vi "Latch.vi"(1 "Reset":bool, 2 "In":bool) -> (0 "Out":bool)   [LabVIEW 2013]
panel:
  in  "var":bool
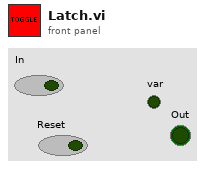
[diagram p1: front panel]
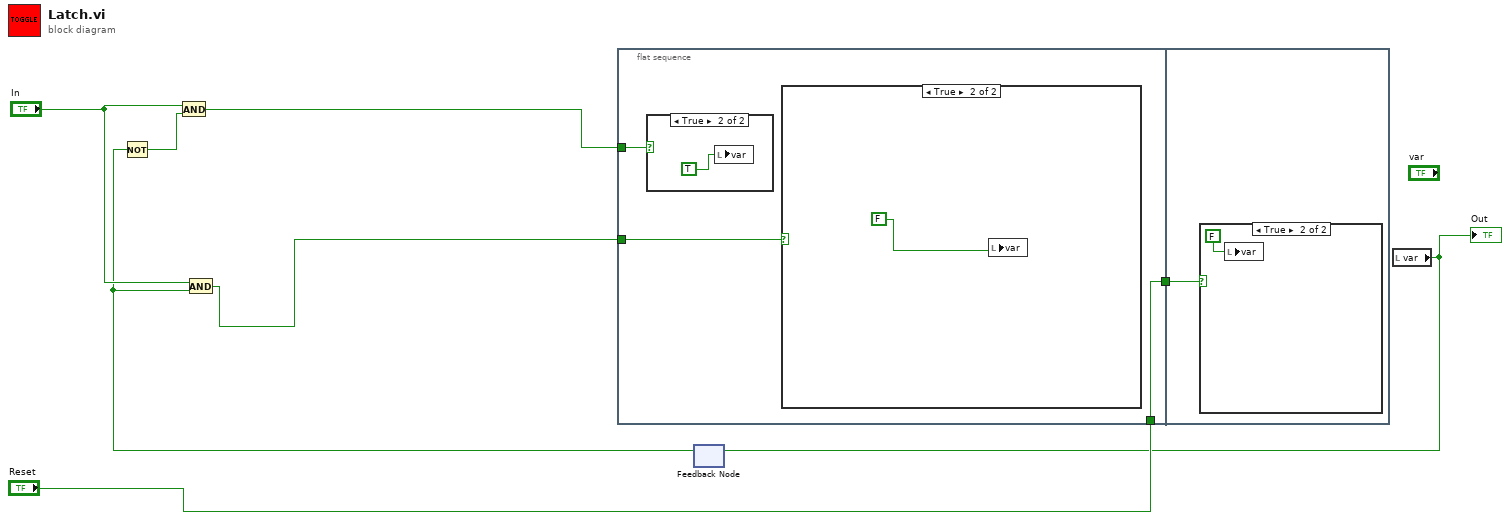
[diagram p0: block diagram]
diagram:
  n1 = flat-sequence {
    tunnel: w6 -> [w11]
    tunnel: w5 -> [w10]
    tunnel: [w9] -> w4
    tunnel: "Reset" -> [w9]
    tunnel: w4 -> [w14]
    frame #0 {
      n2 = case shown="True" w11 {
        frame False {
        }
        frame True {
          n3 = local write "var"(TRUE) -> ()
        }
      }
      n4 = case shown="True" w10 {
        frame False {
        }
        frame True {
          n5 = local write "var"(FALSE) -> ()
        }
      }
    }
    frame #1 {
      n6 = case shown="True" w14 {
        frame False {
        }
        frame True {
          n7 = local write "var"(FALSE) -> ()
        }
      }
    }
  }
  n8 = feedback #1() -> (w2:bool)  [unwired: 1 in]
  n9 = Not(x=w2) -> (.not. x?=w7:bool)
  n10 = And(x="In", y=w7) -> (x .and. y?=w6:bool)
  n11 = And(x="In", y=w2) -> (x .and. y?=w5:bool)
  n12 = local read "var"() -> (w1:bool)
  "Out" <- w1
  n13 = feedback-in #1(w1) -> ()
